vi "main-acq.vi"() -> ()   [LabVIEW 2015]
uses:
  <vilib>/userdefined/High Color/IMAQdx.ctl
  <vilib>/Utility/miscctls.llb/LVPositionTypeDef.ctl
  Global-variables.vi
  <vilib>/vision/driver/NI_Vision_Acquisition_Software.lvlib
  <resource>/objmgr/imaqdx.rc
  <vilib>/vision/NI_Vision_Development_Module.lvlib
panel:
  in  "Tab Control 2":enum32{"Visualization", "Fringe quality map"}(tab)
  out "Camera rigth":T1(plugin-control)
  out "Camera-left":T1(plugin-control)
  out "Camera-left-Map":T1(plugin-control)
  out "Camera-rigth-Map":T1(plugin-control)
  out "Line Profile":dbl[][](graph)
  in  "Stop Button":bool
  in  "Tab Control":T2(tab)
  out "Available?":bool
  in  "Quality map?":bool
  in  "Camera-left":T3="cam4"
  in  "Camera-rigth":T3="cam4"
  in  "Exposure time left":dbl=10000.0
  in  "Exposure time rigth":dbl=10000.0
  out "Available?":bool
  in  "Color background":bool caption="OK Button"
  in  "Central Cross":bool caption="OK Button"
  in  "Central Lines":bool caption="OK Button"
  in  "Intensity":dbl=1.0 min=0.0 max=1.0
  in  "Color background":u32(colorbox)=16448250
  in  "Save Image":bool
  in  "File Format":string(combo)
  in  "Name":string
  in  "Path":path
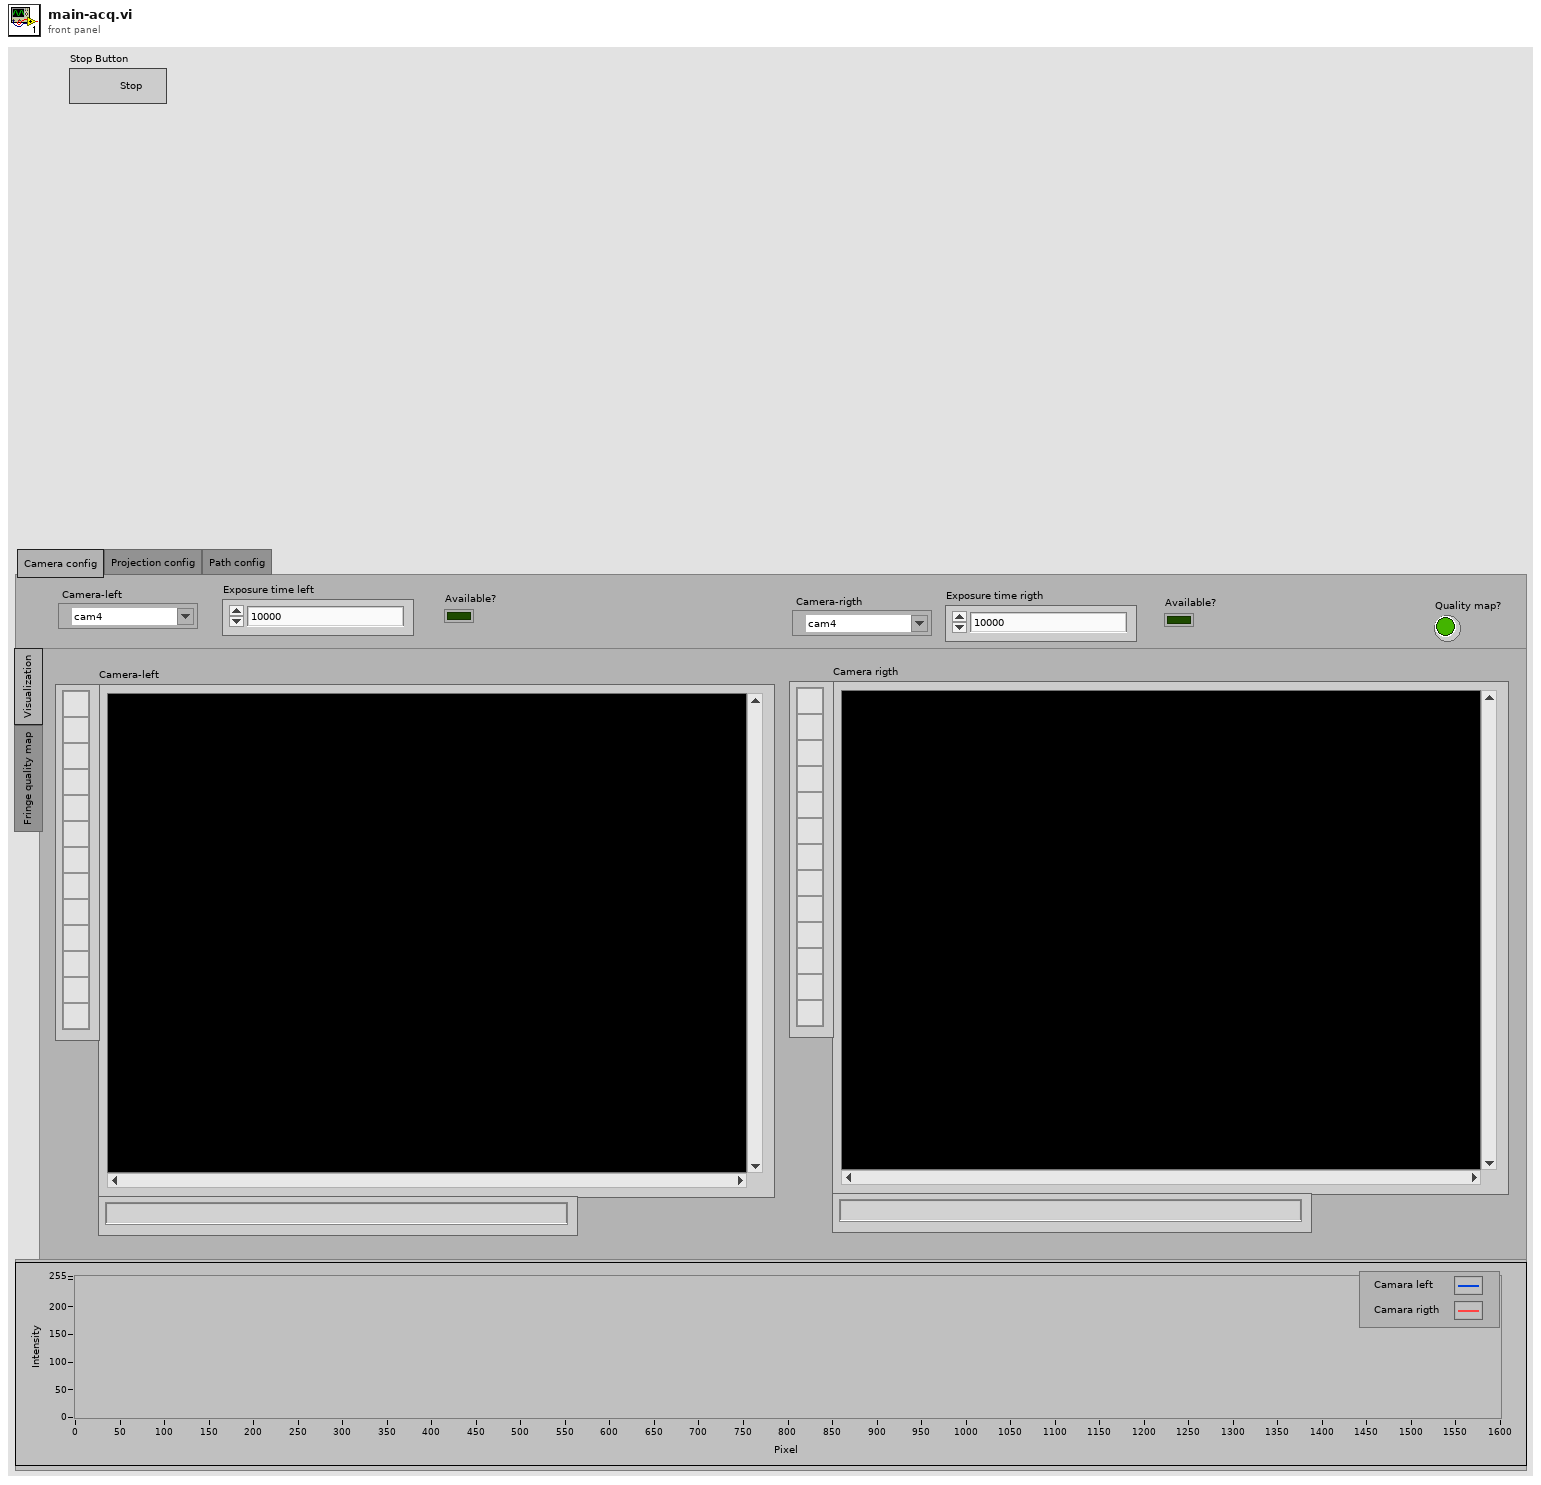
[diagram p1: front panel]
types:
  T1 = typedef "IMAQ Image.ctl" = refnum<image>
  T2 = enum32{"Camera config", "Projection config", "Path config"}
  T3 = typedef "IMAQdx.ctl" = refnum<k21>
  T4 = typedef "LVPositionTypeDef.ctl" = cluster{"Left":i32, "Top":i32}
  T5 = typedef "Image Type" = u32
  T6 = cluster{"Global Rectangle":i32[], "Contours":cluster{"Contour Type":u32, "ROI Type":u32, "Points":i32[]}[]}
  T7 = cluster{"Object Center":cluster{"X":sgl, "Y":sgl}, "Bounding Box":cluster{"X Left":i32, "Y Top":i32, "X Right":i32, "Y Bottom":i32}, "Area":sgl, "Orientation":sgl, "Aspect Ratio":sgl, "Nb Holes":i32}[]
  T8 = typedef "LVAllMonitorsDisplayTypeDef.ctl" = cluster{"Bounds":cluster{"Left":i16, "Top":i16, "Right":i16, "Bottom":i16}, "Depth":i16}[]
  T9 = cluster{"Bounds":cluster{"Left":i16, "Top":i16, "Right":i16, "Bottom":i16}, "Depth":i16}
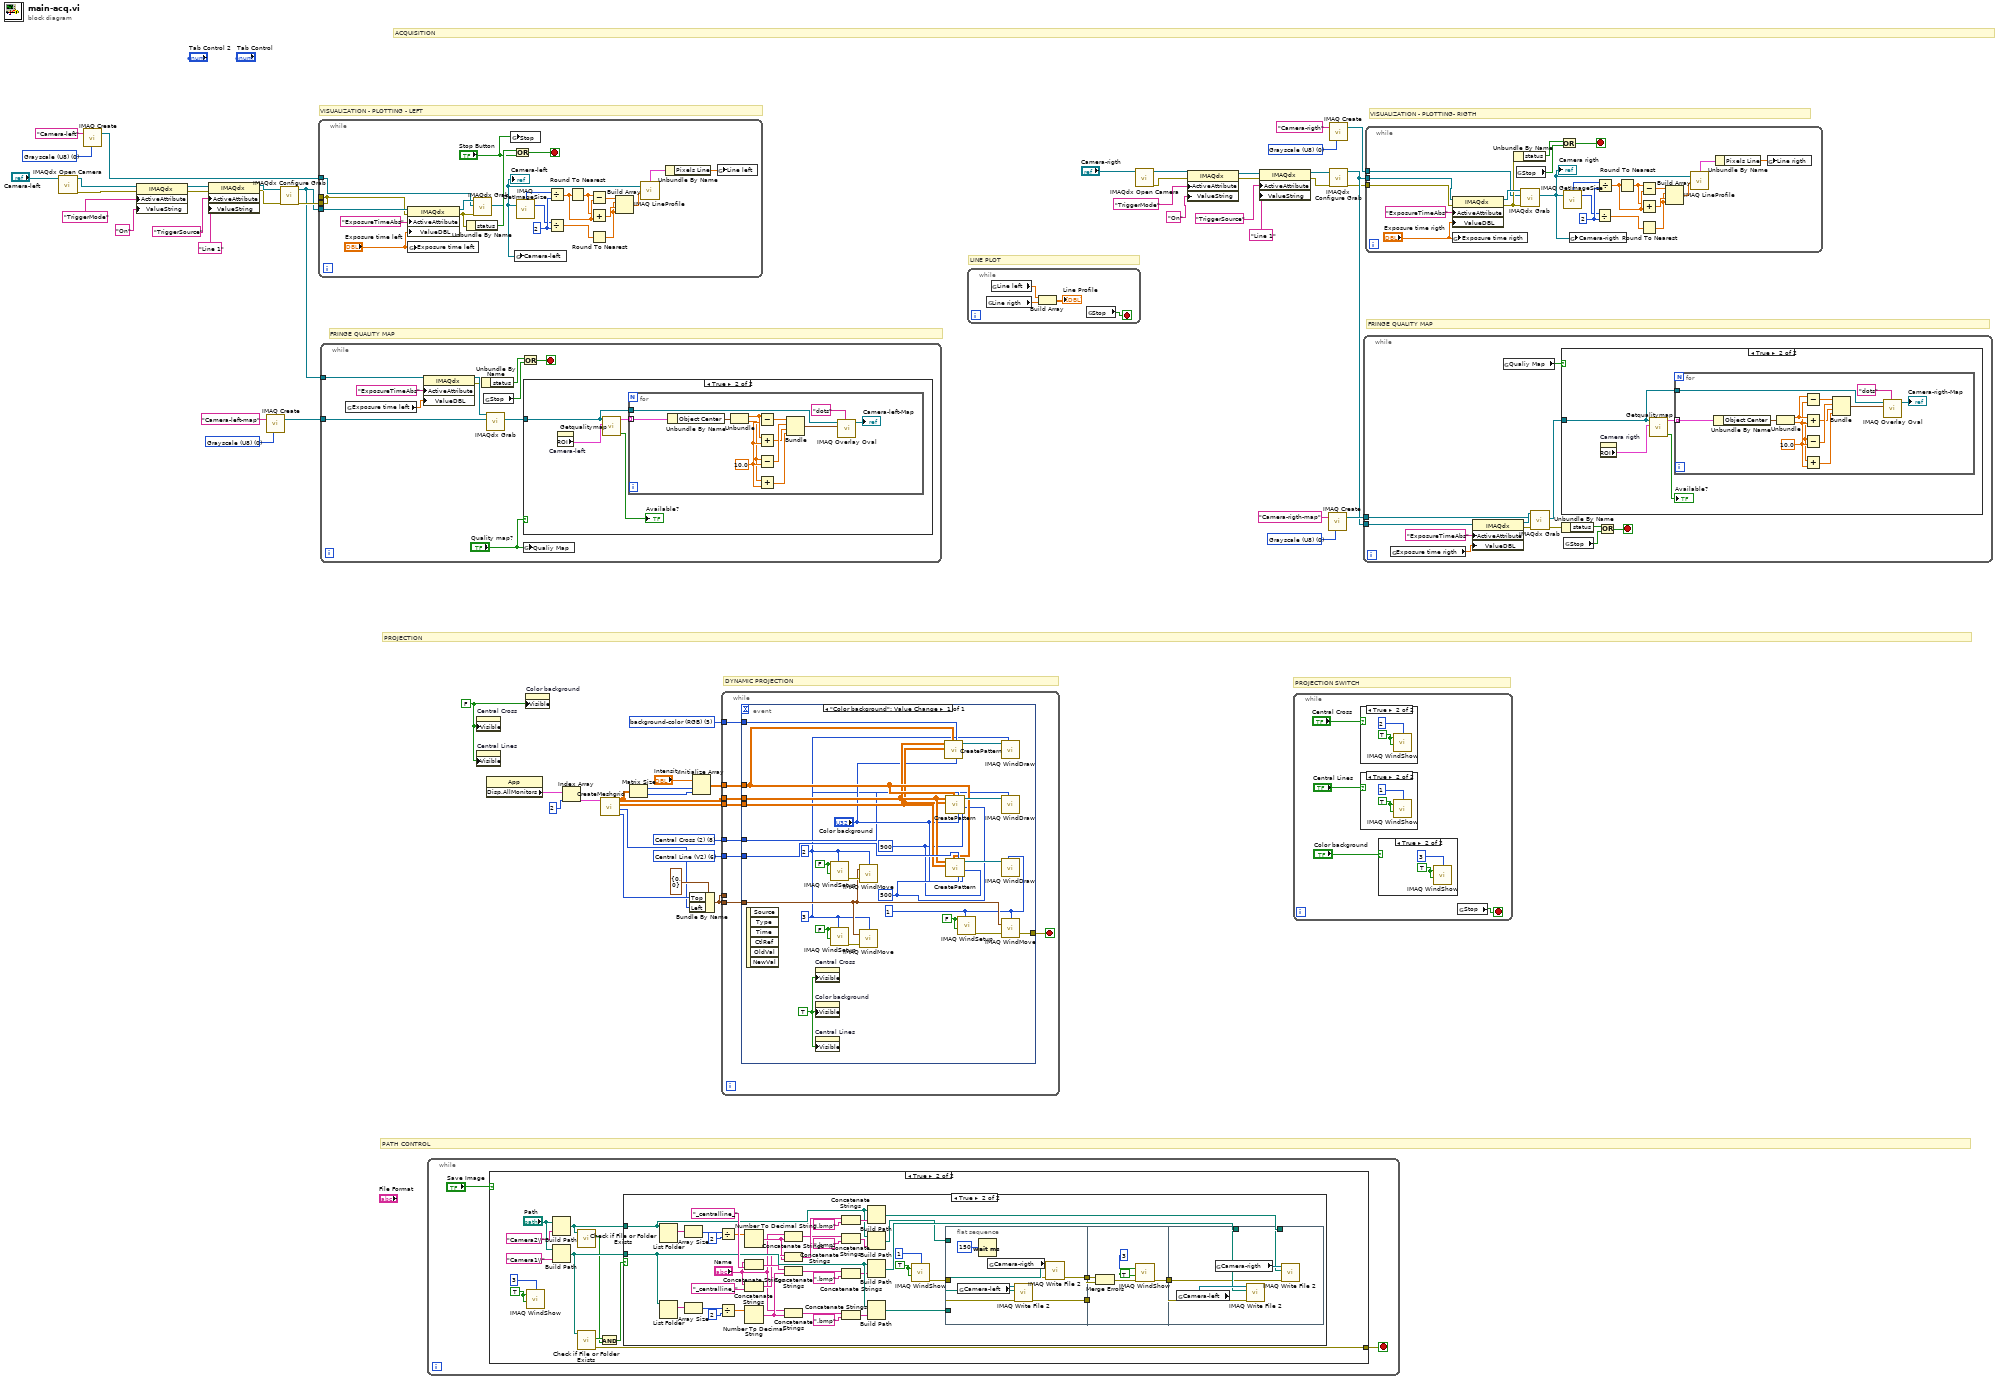
[diagram p0: block diagram]
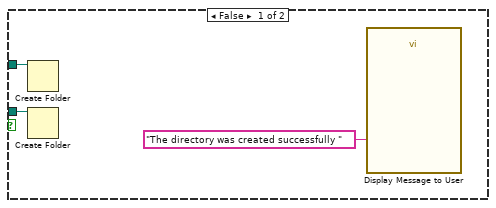
[diagram p3: hidden frame]
diagram:
  w27 = FALSE
  w28 = T5 8 items=["Fringes Pattern (V)", "Fringes Pattern (H)", "Central Line (V)", "Central Line (H)", "Central Cross", "background-color (RGB)", "Central Line (V2)", "Central Line (H2)", "Central Cross (2)"] ("Image Type")
  w29 = T5 6 items=["Fringes Pattern (V)", "Fringes Pattern (H)", "Central Line (V)", "Central Line (H)", "Central Cross", "background-color (RGB)", "Central Line (V2)", "Central Line (H2)", "Central Cross (2)"] ("Image Type")
  w33 = T5 5 items=["Fringes Pattern (V)", "Fringes Pattern (H)", "Central Line (V)", "Central Line (H)", "Central Cross", "background-color (RGB)", "Central Line (V2)", "Central Line (H2)", "Central Cross (2)"] ("Image Type")
  w43 = T5 0 items=["Grayscale (U8)", "Grayscale (I16)", "Grayscale (SGL)", "Complex (CSG)", "RGB (U32)", "HSL (U32)", "RGB (U64)"] ("Image Type")
  w49 = T5 0 items=["Grayscale (U8)", "Grayscale (I16)", "Grayscale (SGL)", "Complex (CSG)", "RGB (U32)", "HSL (U32)", "RGB (U64)"] ("Image Type")
  w52 = T5 0 items=["Grayscale (U8)", "Grayscale (I16)", "Grayscale (SGL)", "Complex (CSG)", "RGB (U32)", "HSL (U32)", "RGB (U64)"] ("Image Type")
  w53 = T5 0 items=["Grayscale (U8)", "Grayscale (I16)", "Grayscale (SGL)", "Complex (CSG)", "RGB (U32)", "HSL (U32)", "RGB (U64)"] ("Image Type")
  # "PATH CONTROL"
  # "PROJECTION SWITCH"
  # "DYNAMIC PROJECTION"
  # "PROJECTION"
  # "ACQUISITION"
  # "FRINGE QUALITY MAP"
  # "LINE PLOT"
  # "FRINGE QUALITY MAP"
  # "VISUALIZATION - PLOTTING- RIGTH"
  # "VISUALIZATION - PLOTTING - LEFT"
  n1 = call <vilib>:"IMAQdx Open Camera.vi"("Session In"="Camera-left") -> ("error out"=w15:errorcluster, "Session Out"=w16:T3)  [unwired: 2 in, 7 out]
  n2 = call "IMAQ Create"("Image Name"="Camera-left", "Image Type"=w52) -> ("New Image"=w50:T1)  [unwired: 2 in, 2 out]
  n3 = property on="Property Node left" class="IMAQdx"(reference=w16, error in=w15, "ActiveAttribute"="TriggerMode" ("String"), "ValueString"="On") -> (reference out=w20:T3, error out=w19:errorcluster)
  n4 = property on="Property Node left" class="IMAQdx"(reference=w20, error in=w19, "ActiveAttribute"="TriggerSource" ("String"), "ValueString"="Line 1") -> (reference out=w14:T3, error out=w13:errorcluster)
  n5 = call "IMAQ Create"("Image Name"="Camera-left-map", "Image Type"=w49) -> ("New Image"=w47:T1)  [unwired: 2 in, 2 out]
  n6 = call <vilib>:"IMAQdx Configure Grab.vi"("error in"=w13, "Session In"=w14) -> ("error out"=w12:errorcluster, "Session Out"=w11:T3)  [unwired: 8 out]
  n7 = while {
    tunnel: w50 -> [w76]
    tunnel: w11 -> [w57]
    tunnel: [w56] -> _
    tunnel: w12 -> [w56]
    stop <- w62 stop-if-true
    w72 = 2
    n8 = property on="Property Node left" class="IMAQdx"(reference=w57, error in=w56, "ActiveAttribute"="ExposureTimeAbs" ("String"), "ValueDBL"="Exposure time left") -> (reference out=w77:T3, error out=w61:errorcluster)
    n9 = global write "Global-variables.vi" "Exposure time left"("Exposure time left") -> ()
    n10 = Unbundle By Name(w61) -> ("status"=w64:bool)
    n11 = call <vilib>:"IMAQdx Grab.vi"("error in"=w61, "Image In"=w76, "Session In"=w77) -> ("Image Out"=w58:T1)  [unwired: 1 in, 7 out]
    "Camera-left" <- w58
    n12 = global write "Global-variables.vi" "Stop"("Stop Button") -> ()
    n13 = Or(x=w64, y="Stop Button") -> (x .or. y?=w62:bool)
    n14 = global write "Global-variables.vi" "Camera-left"(w58) -> ()
    n15 = call "IMAQ GetImageSize"("Image"=w58) -> ("Y Resolution"=w71:i32, "X Resolution"=w70:i32)  [unwired: 3 in, 1 out]
    n16 = Divide(x=w70, y=w72) -> (x/y=w75:dbl)
    n17 = Divide(x=w71, y=w72) -> (x/y=w74:dbl)
    n18 = Round To Nearest(number=w75) -> (nearest integer value=w73:dbl)
    n19 = Subtract(x=w73, y=w75) -> (x-y=w69:dbl)
    n20 = Add(x=w73, y=w75) -> (x+y=w68:dbl)
    n21 = Round To Nearest(number=w74) -> (nearest integer value=w67:dbl)
    n22 = Build Array(w69, w67, w68, w67) -> (w65:dbl[])
    n23 = call "IMAQ LineProfile"("Line Coordinates"=w65, "Image"=w58) -> ("Line Graph"=w66:cluster{"x0":sgl, "dx":sgl, "Pixels Line":sgl[]})  [unwired: 1 in, 5 out]
    n24 = Unbundle By Name(w66) -> ("Pixels Line"=w59:sgl[])
    n25 = global write "Global-variables.vi" "Line left"(w59) -> ()
  }
  n26 = while {
    tunnel: w47 -> [w84]
    tunnel: w11 -> [w81]
    stop <- w89 stop-if-true
    n27 = global read "Global-variables.vi" "Exposure time left"() -> (w86:dbl)
    n28 = property on="Property Node left-map" class="IMAQdx"(reference=w81, "ActiveAttribute"="ExposureTimeAbs" ("String"), "ValueDBL"=w86) -> (reference out=w85:T3, error out=w83:errorcluster)  [unwired: 1 in]
    n29 = Unbundle By Name(w83) -> ("status"=w82:bool)
    n30 = global read "Global-variables.vi" "Stop"() -> (w88:bool)
    n31 = call <vilib>:"IMAQdx Grab.vi"("Image In"=w84, "Session In"=w85) -> ("Image Out"=w79:T1)  [unwired: 2 in, 7 out]
    n32 = Or(x=w82, y=w88) -> (x .or. y?=w89:bool)
    n33 = case shown="True" "Quality map?" {
      tunnel: w79 -> [_ w92]
      frame False {
      }
      frame True {
        n34 = property on="Camera-left" class="ImageControl"() -> ("ROI"=w91:T6)  [unwired: 2 in, 2 out]
        n35 = call "Getqualitymap.vi"("ROI"=w91, "Refnum in"=w92) -> ("x != 0?"=→"Available?":bool, "Objects"=w93:T7)  [unwired: 7 in, 1 out]
        n36 = for {
          tunnel: w92 -> [w95]
          tunnel: w93 -> [w96] mode=indexing
          w100 = 10.0
          n37 = Unbundle By Name(w96) -> ("Object Center"=w106:cluster{"X":sgl, "Y":sgl})
          n38 = Unbundle(w106) -> ("X"=w101:sgl, "Y"=w99:sgl)
          n39 = Subtract(x=w101, y=w100) -> (x-y=w105:dbl)
          n40 = Add(x=w101, y=w100) -> (x+y=w103:dbl)
          n41 = Subtract(x=w99, y=w100) -> (x-y=w104:dbl)
          n42 = Add(x=w99, y=w100) -> (x+y=w102:dbl)
          n43 = Bundle(w105, w104, w103, w102) -> (w97:cluster{dbl, dbl, dbl, dbl})  [unwired: 1 in]
          n44 = call "IMAQ Overlay Oval"("Group"="dots", "Bounding Rectangle"=w97, "Image"=w95) -> ("Image Out"=→"Camera-left-Map":T1)  [unwired: 7 in, 1 out]
        }
      }
    }
    n45 = global write "Global-variables.vi" "Qualiy Map"("Quality map?") -> ()
  }
  n46 = while {
    stop <- w107 stop-if-true
    n47 = case shown="True" "Save Image" {
      tunnel: [_ w117] -> w107
      frame False {
      }
      frame True {
        w110 = TRUE
        n48 = call "IMAQ WindShow"("Bring To Front? (N)"=w110, "Hide/Show (Show)"=w110, "Window Number (0...15)"=3) -> ()  [unwired: 3 in, 3 out]
        n49 = Build Path(base path="Path", name or relative path="Camera2\\") -> (appended path=w111:path)
        n50 = Build Path(base path="Path", name or relative path="Camera1\\") -> (appended path=w118:path)
        n51 = call <vilib>:"Check if File or Folder Exists.vi"("path"=w111) -> ("file or folder exists?"=w113:bool)  [unwired: 8 in, 2 out]
        n52 = call <vilib>:"Check if File or Folder Exists.vi"("path"=w118) -> ("error out"=w117:errorcluster, "file or folder exists?"=w114:bool)  [unwired: 8 in, 1 out]
        n53 = And(x=w114, y=w113) -> (x .and. y?=w112:bool)
        n54 = case shown="True" w112 {
          tunnel: w118 -> [w122 w154]
          tunnel: w111 -> [w121 w130]
          frame False {
            n55 = Create Folder(path (use dialog)=w121) -> ()  [unwired: 2 in, 3 out]
            n56 = Create Folder(path (use dialog)=w122) -> ()  [unwired: 2 in, 3 out]
            n57 = call "Display Message to User"("Message"="The directory was created successfully ") -> ()  [unwired: 9 in, 2 out]
          }
          frame True {
            w124 = TRUE
            n58 = List Folder(path=w130) -> (filenames=w143:string[])  [unwired: 3 in, 3 out]
            n59 = List Folder(path=w154) -> (filenames=w161:string[])  [unwired: 3 in, 3 out]
            n60 = Array Size(array=w143) -> (size(s)=w142:i32)
            n61 = Array Size(array=w161) -> (size(s)=w160:i32)
            n62 = Divide(x=w142, y=2) -> (x/y=w140:dbl)
            n63 = Divide(x=w160, y=2) -> (x/y=w158:dbl)
            n64 = Number To Decimal String(number=w140) -> (decimal integer string=w137:string)  [unwired: 1 in]
            n65 = Concatenate Strings("Name", "_centralline_") -> (w156:string)
            n66 = Concatenate Strings("Name", "_centralline_") -> (w138:string)
            n67 = Number To Decimal String(number=w158) -> (decimal integer string=w155:string)  [unwired: 1 in]
            n68 = Concatenate Strings("Name", w137) -> (w133:string)
            n69 = Concatenate Strings(w138, w137) -> (w136:string)
            n70 = Concatenate Strings(w156, w155) -> (w153:string)
            n71 = Concatenate Strings("Name", w155) -> (w150:string)
            n72 = Concatenate Strings(w136, ".bmp") -> (w134:string)
            n73 = Concatenate Strings(w133, ".bmp") -> (w131:string)
            n74 = Concatenate Strings(w153, ".bmp") -> (w151:string)
            n75 = Concatenate Strings(w150, ".bmp") -> (w148:string)
            n76 = Build Path(base path=w130, name or relative path=w134) -> (appended path=w127:path)
            n77 = Build Path(base path=w130, name or relative path=w131) -> (appended path=w128:path)
            n78 = Build Path(base path=w154, name or relative path=w151) -> (appended path=w147:path)
            n79 = Build Path(base path=w154, name or relative path=w148) -> (appended path=w146:path)
            n80 = call "IMAQ WindShow"("Bring To Front? (N)"=w124, "Hide/Show (Show)"=w124, "Window Number (0...15)"=1) -> ("error out"=w123:errorcluster)  [unwired: 3 in, 2 out]
            n81 = flat-sequence {
              tunnel: w146 -> [w168]
              tunnel: w128 -> [w166]
              tunnel: [w165] -> w126
              tunnel: [w164] -> w125
              tunnel: w123 -> [w163]
              tunnel: [w173] -> w144
              tunnel: w126 -> [w172]
              tunnel: w125 -> [w171]
              tunnel: w147 -> [w179]
              tunnel: w144 -> [w176]
              tunnel: w127 -> [w177]
              frame #0 {
                n82 = global read "Global-variables.vi" "Camera-left"() -> (w169:T1)
                n83 = Wait (ms)(milliseconds to wait=150) -> ()  [unwired: 1 out]
                n84 = global read "Global-variables.vi" "Camera-rigth"() -> (w167:T1)
                n85 = call-poly "IMAQ Write File 2"("error in (no error)"=w163, "File Path"=w168, "Image"=w169) -> ("error out"=w164:errorcluster)  [unwired: 7 in, 1 out]
                n86 = call-poly "IMAQ Write File 2"("error in (no error)"=w163, "File Path"=w166, "Image"=w167) -> ("error out"=w165:errorcluster)  [unwired: 7 in, 1 out]
              }
              frame #1 {
                w175 = TRUE
                n87 = Merge Errors(w172, w171) -> (w170:errorcluster)
                n88 = call "IMAQ WindShow"("error in (no error)"=w170, "Bring To Front? (N)"=w175, "Hide/Show (Show)"=w175, "Window Number (0...15)"=3) -> ("error out"=w173:errorcluster)  [unwired: 2 in, 2 out]
              }
              frame #2 {
                n89 = global read "Global-variables.vi" "Camera-left"() -> (w180:T1)
                n90 = global read "Global-variables.vi" "Camera-rigth"() -> (w178:T1)
                n91 = call-poly "IMAQ Write File 2"("error in (no error)"=w176, "File Path"=w179, "Image"=w180) -> ()  [unwired: 7 in, 2 out]
                n92 = call-poly "IMAQ Write File 2"("error in (no error)"=w176, "File Path"=w177, "Image"=w178) -> ()  [unwired: 7 in, 2 out]
              }
            }
          }
        }
      }
    }
  }
  n93 = property on="Central Cross" class="Bool (strict)"("Visible"=w27) -> ()  [unwired: 2 in, 2 out]
  n94 = property on="Central Lines" class="Bool (strict)"("Visible"=w27) -> ()  [unwired: 2 in, 2 out]
  n95 = property class="App"() -> ("Disp.AllMonitors"=w35:T8)  [unwired: 2 in, 2 out]
  n96 = property on="Color background" class="Bool (strict)"("Visible"=w27) -> ()  [unwired: 2 in, 2 out]
  n97 = Index Array(array=w35, index=2) -> (element=w39:T9)
  n98 = call "CreateMeshgrid.vi"("Cluster"=w39) -> ("Top"=w25:i32, "Left"=w24:i32, "Y"=w30:dbl[][], "X"=w31:dbl[][])  [unwired: 7 in]
  n99 = Matrix Size(0:w31) -> (1:w37:i32, 2:w36:i32)
  n100 = Bundle By Name(cluster=T4 {"Left"=0, "Top"=0} ("Position"), "Top"=w25, "Left"=w24) -> (w23:T4)
  n101 = Initialize Array("Intensity", w37, w36) -> (w32:dbl[][])
  n102 = while {
    tunnel: w33 -> [w187]
    tunnel: w32 -> [w186]
    tunnel: w31 -> [w185]
    tunnel: w30 -> [w184]
    tunnel: w29 -> [w183]
    tunnel: w28 -> [w182]
    tunnel: w23 -> [w181]
    tunnel: w23 -> [_]
    stop <- w188 stop-if-true
    n103 = event shown="[0] \"Color background\": Value Change" {
      selector: _ -> [_]
      dyn-events: _ -> [_]
      timeout: _ -> [_]
      tunnel: [w210] -> w188
      tunnel: w187 -> [w209]
      tunnel: w186 -> [w200]
      tunnel: w185 -> [w199]
      tunnel: w184 -> [w198]
      tunnel: w183 -> [w204]
      tunnel: w182 -> [w196]
      tunnel: w181 -> [w194]
      event "Color background": Value Change {
        w192 = 900
        w193 = 500
        w195 = TRUE
        w203 = FALSE
        w190 = 3
        w207 = FALSE
        w191 = 2
        w212 = FALSE
        w189 = 1
        n104 = event-data() -> ()  [unwired: 1 in, 6 out]
        n105 = property on="Central Cross" class="Bool (strict)"("Visible"=w195) -> ()  [unwired: 2 in, 2 out]
        n106 = property on="Color background" class="Bool (strict)"("Visible"=w195) -> ()  [unwired: 2 in, 2 out]
        n107 = property on="Central Lines" class="Bool (strict)"("Visible"=w195) -> ()  [unwired: 2 in, 2 out]
        n108 = call "IMAQ WindSetup"("Window Number (0...15)"=w191, "Window has title bar? (Yes)"=w207, "Window can grow? (Yes)"=w207) -> ("error out"=w206:errorcluster)  [unwired: 8 in]
        n109 = call "IMAQ WindSetup"("Window Number (0...15)"=w190, "Window has title bar? (Yes)"=w203, "Window can grow? (Yes)"=w203) -> ("error out"=w202:errorcluster)  [unwired: 8 in]
        n110 = call "IMAQ WindMove"("Window Number (0...15)"=w191, "Coordinates (screen)"=w194, "error in (no error)"=w206) -> ()  [unwired: 2 in, 2 out]
        n111 = call "IMAQ WindMove"("Window Number (0...15)"=w190, "Coordinates (screen)"=w194, "error in (no error)"=w202) -> ()  [unwired: 2 in, 2 out]
        n112 = call "CreatePattern.vi"("Color Box"="Color background", "Pattern Type"=w209, "Intensity"=w200, "Y"=w198, "X"=w199) -> ("Refnum out"=w208:T1)  [unwired: 5 in, 1 out]
        n113 = call "CreatePattern.vi"("Coord-2"=w192, "Coord-1"=w193, "Color Box"="Color background", "Pattern Type"=w196, "Intensity"=w200, "Y"=w198, "X"=w199) -> ("Refnum out"=w201:T1)  [unwired: 3 in, 1 out]
        n114 = call "CreatePattern.vi"("Coord-2"=w193, "Coord-1"=w192, "Color Box"="Color background", "Pattern Type"=w204, "Intensity"=w200, "Y"=w198, "X"=w199) -> ("Refnum out"=w205:T1)  [unwired: 3 in, 1 out]
        n115 = call "IMAQ WindSetup"("Window Number (0...15)"=w189, "Window has title bar? (Yes)"=w212, "Window can grow? (Yes)"=w212) -> ("error out"=w211:errorcluster)  [unwired: 8 in]
        n116 = call "IMAQ WindDraw"("Window Number (0...15)"=w190, "Image"=w208) -> ()  [unwired: 8 in, 2 out]
        n117 = call "IMAQ WindDraw"("Window Number (0...15)"=w191, "Image"=w201) -> ()  [unwired: 8 in, 2 out]
        n118 = call "IMAQ WindDraw"("Window Number (0...15)"=w189, "Image"=w205) -> ()  [unwired: 8 in, 2 out]
        n119 = call "IMAQ WindMove"("Window Number (0...15)"=w189, "Coordinates (screen)"=w194, "error in (no error)"=w211) -> ("error out"=w210:errorcluster)  [unwired: 2 in, 1 out]
      }
    }
  }
  n120 = while {
    stop <- w216 stop-if-true
    n121 = global read "Global-variables.vi" "Line rigth"() -> (w214:dbl[])
    n122 = global read "Global-variables.vi" "Line left"() -> (w215:dbl[])
    n123 = Build Array(w215, w214) -> (→"Line Profile":dbl[][])
    n124 = global read "Global-variables.vi" "Stop"() -> (w216:bool)
  }
  n125 = call <vilib>:"IMAQdx Open Camera.vi"("Session In"="Camera-rigth") -> ("error out"=w4:errorcluster, "Session Out"=w5:T3)  [unwired: 2 in, 7 out]
  n126 = property on="Property Node left" class="IMAQdx"(reference=w5, error in=w4, "ActiveAttribute"="TriggerMode" ("String"), "ValueString"="On") -> (reference out=w9:T3, error out=w8:errorcluster)
  n127 = property on="Property Node left" class="IMAQdx"(reference=w9, error in=w8, "ActiveAttribute"="TriggerSource" ("String"), "ValueString"="Line 1") -> (reference out=w3:T3, error out=w2:errorcluster)
  n128 = while {
    stop <- w217 stop-if-true
    n129 = case shown="True" "Central Cross" {
      frame False {
      }
      frame True {
        w223 = TRUE
        n130 = call "IMAQ WindShow"("Bring To Front? (N)"=w223, "Hide/Show (Show)"=w223, "Window Number (0...15)"=2) -> ()  [unwired: 3 in, 3 out]
      }
    }
    n131 = case shown="True" "Central Lines" {
      frame False {
      }
      frame True {
        w225 = TRUE
        n132 = call "IMAQ WindShow"("Bring To Front? (N)"=w225, "Hide/Show (Show)"=w225, "Window Number (0...15)"=1) -> ()  [unwired: 3 in, 3 out]
      }
    }
    n133 = case shown="True" "Color background" {
      frame False {
      }
      frame True {
        w221 = TRUE
        n134 = call "IMAQ WindShow"("Bring To Front? (N)"=w221, "Hide/Show (Show)"=w221, "Window Number (0...15)"=3) -> ()  [unwired: 3 in, 3 out]
      }
    }
    n135 = global read "Global-variables.vi" "Stop"() -> (w217:bool)
  }
  n136 = call "IMAQ Create"("Image Name"="Camera-rigth-map", "Image Type"=w43) -> ("New Image"=w42:T1)  [unwired: 2 in, 2 out]
  n137 = call "IMAQ Create"("Image Name"="Camera-rigth", "Image Type"=w53) -> ("New Image"=w45:T1)  [unwired: 2 in, 2 out]
  n138 = call <vilib>:"IMAQdx Configure Grab.vi"("error in"=w2, "Session In"=w3) -> ("error out"=w40:errorcluster, "Session Out"=w41:T3)  [unwired: 8 out]
  n139 = while {
    tunnel: w42 -> [w235]
    tunnel: w41 -> [w229]
    stop <- w230 stop-if-true
    n140 = global read "Global-variables.vi" "Exposure time rigth"() -> (w237:dbl)
    n141 = property on="Property Node rigth" class="IMAQdx"(reference=w229, "ActiveAttribute"="ExposureTimeAbs" ("String"), "ValueDBL"=w237) -> (reference out=w236:T3, error out=w234:errorcluster)  [unwired: 1 in]
    n142 = global read "Global-variables.vi" "Qualiy Map"() -> (w227:bool)
    n143 = call <vilib>:"IMAQdx Grab.vi"("error in"=w234, "Image In"=w235, "Session In"=w236) -> ("error out"=w231:errorcluster, "Image Out"=w228:T1)  [unwired: 1 in, 6 out]
    n144 = case shown="True" w227 {
      tunnel: w228 -> [_ w241]
      frame False {
      }
      frame True {
        n145 = property on="Camera rigth" class="ImageControl"() -> ("ROI"=w240:T6)  [unwired: 2 in, 2 out]
        n146 = call "Getqualitymap.vi"("ROI"=w240, "Refnum in"=w241) -> ("x != 0?"=→"Available?":bool, "Objects"=w242:T7)  [unwired: 7 in, 1 out]
        n147 = for {
          tunnel: w242 -> [w244] mode=indexing
          tunnel: w241 -> [w243]
          w249 = 10.0
          n148 = Unbundle By Name(w244) -> ("Object Center"=w255:cluster{"X":sgl, "Y":sgl})
          n149 = Unbundle(w255) -> ("X"=w250:sgl, "Y"=w248:sgl)
          n150 = Subtract(x=w250, y=w249) -> (x-y=w254:dbl)
          n151 = Add(x=w250, y=w249) -> (x+y=w252:dbl)
          n152 = Subtract(x=w248, y=w249) -> (x-y=w253:dbl)
          n153 = Add(x=w248, y=w249) -> (x+y=w251:dbl)
          n154 = Bundle(w254, w253, w252, w251) -> (w246:cluster{dbl, dbl, dbl, dbl})  [unwired: 1 in]
          n155 = call "IMAQ Overlay Oval"("Group"="dots", "Bounding Rectangle"=w246, "Image"=w243) -> ("Image Out"=→"Camera-rigth-Map":T1)  [unwired: 7 in, 1 out]
        }
      }
    }
    n156 = Unbundle By Name(w231) -> ("status"=w233:bool)
    n157 = global read "Global-variables.vi" "Stop"() -> (w232:bool)
    n158 = Or(x=w233, y=w232) -> (x .or. y?=w230:bool)
  }
  n159 = while {
    tunnel: w41 -> [w276]
    tunnel: w40 -> [w275]
    tunnel: w45 -> [w258]
    stop <- w273 stop-if-true
    w267 = 2
    n160 = property on="Property Node rigth" class="IMAQdx"(reference=w276, error in=w275, "ActiveAttribute"="ExposureTimeAbs" ("String"), "ValueDBL"="Exposure time rigth") -> (reference out=w277:T3, error out=w274:errorcluster)
    n161 = global write "Global-variables.vi" "Exposure time rigth"("Exposure time rigth") -> ()
    n162 = Unbundle By Name(w274) -> ("status"=w272:bool)
    n163 = global read "Global-variables.vi" "Stop"() -> (w271:bool)
    n164 = call <vilib>:"IMAQdx Grab.vi"("error in"=w274, "Image In"=w258, "Session In"=w277) -> ("Image Out"=w256:T1)  [unwired: 1 in, 7 out]
    "Camera rigth" <- w256
    n165 = Or(x=w272, y=w271) -> (x .or. y?=w273:bool)
    n166 = call "IMAQ GetImageSize"("Image"=w256) -> ("Y Resolution"=w266:i32, "X Resolution"=w265:i32)  [unwired: 3 in, 1 out]
    n167 = global write "Global-variables.vi" "Camera-rigth"(w256) -> ()
    n168 = Divide(x=w266, y=w267) -> (x/y=w269:dbl)
    n169 = Divide(x=w265, y=w267) -> (x/y=w270:dbl)
    n170 = Round To Nearest(number=w270) -> (nearest integer value=w268:dbl)
    n171 = Subtract(x=w268, y=w270) -> (x-y=w264:dbl)
    n172 = Add(x=w268, y=w270) -> (x+y=w263:dbl)
    n173 = Round To Nearest(number=w269) -> (nearest integer value=w262:dbl)
    n174 = Build Array(w264, w262, w263, w262) -> (w260:dbl[])
    n175 = call "IMAQ LineProfile"("Line Coordinates"=w260, "Image"=w256) -> ("Line Graph"=w261:cluster{"x0":sgl, "dx":sgl, "Pixels Line":sgl[]})  [unwired: 1 in, 5 out]
    n176 = Unbundle By Name(w261) -> ("Pixels Line"=w259:sgl[])
    n177 = global write "Global-variables.vi" "Line rigth"(w259) -> ()
  }
